vi "压力判定.vi"(7 "Result":refnum<vi>, 10 "判定参数":T2, 11 "XY曲线":cluster{"X":dbl[], "Y":dbl[]}[](array[cluster])) -> (2 "大小":i32, 3 "OK？":bool)   [LabVIEW 2020]
uses:
  Global_Variable/Global.vi
panel:
  in  "最大值判定":T1
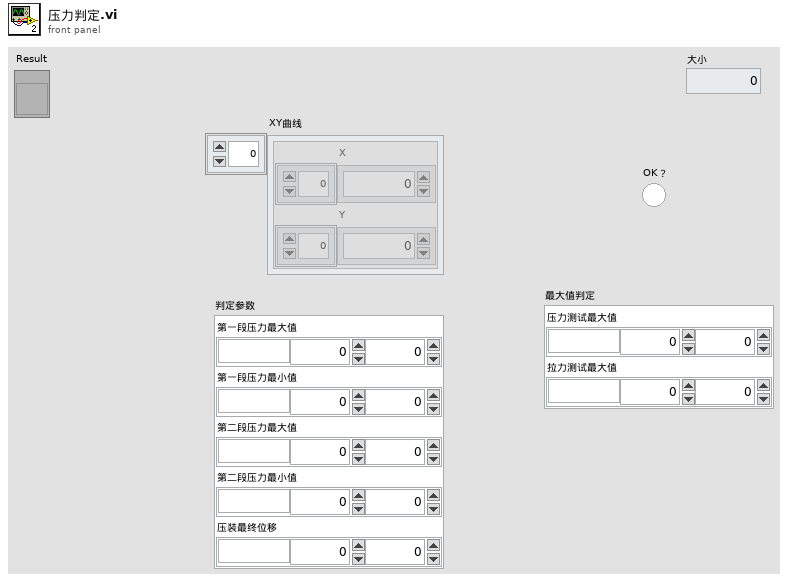
[diagram p1: front panel]
types:
  T1 = cluster{"压力测试最大值":cluster{"单位":string, "下限":dbl, "上限":dbl}, "拉力测试最大值":cluster{"单位":string, "下限":dbl, "上限":dbl}}
  T2 = cluster{"第一段压力最大值":cluster{"单位":string, "下限":dbl, "上限":dbl}, "第一段压力最小值":cluster{"单位":string, "下限":dbl, "上限":dbl}, "第二段压力最大值":cluster{"单位":string, "下限":dbl, "上限":dbl}, "第二段压力最小值":cluster{"单位":string, "下限":dbl, "上限":dbl}, "压装最终位移":cluster{"单位":string, "下限":dbl, "上限":dbl}}
  T3 = cluster{"第一段判定框位移":cluster{"单位":string, "下限":dbl, "上限":dbl}, "第一段判定框压力":cluster{"单位":string, "下限":dbl, "上限":dbl}, "低二段判定框位移":cluster{"单位":string, "下限":dbl, "上限":dbl}, "第二段判定框压力":cluster{"单位":string, "下限":dbl, "上限":dbl}}
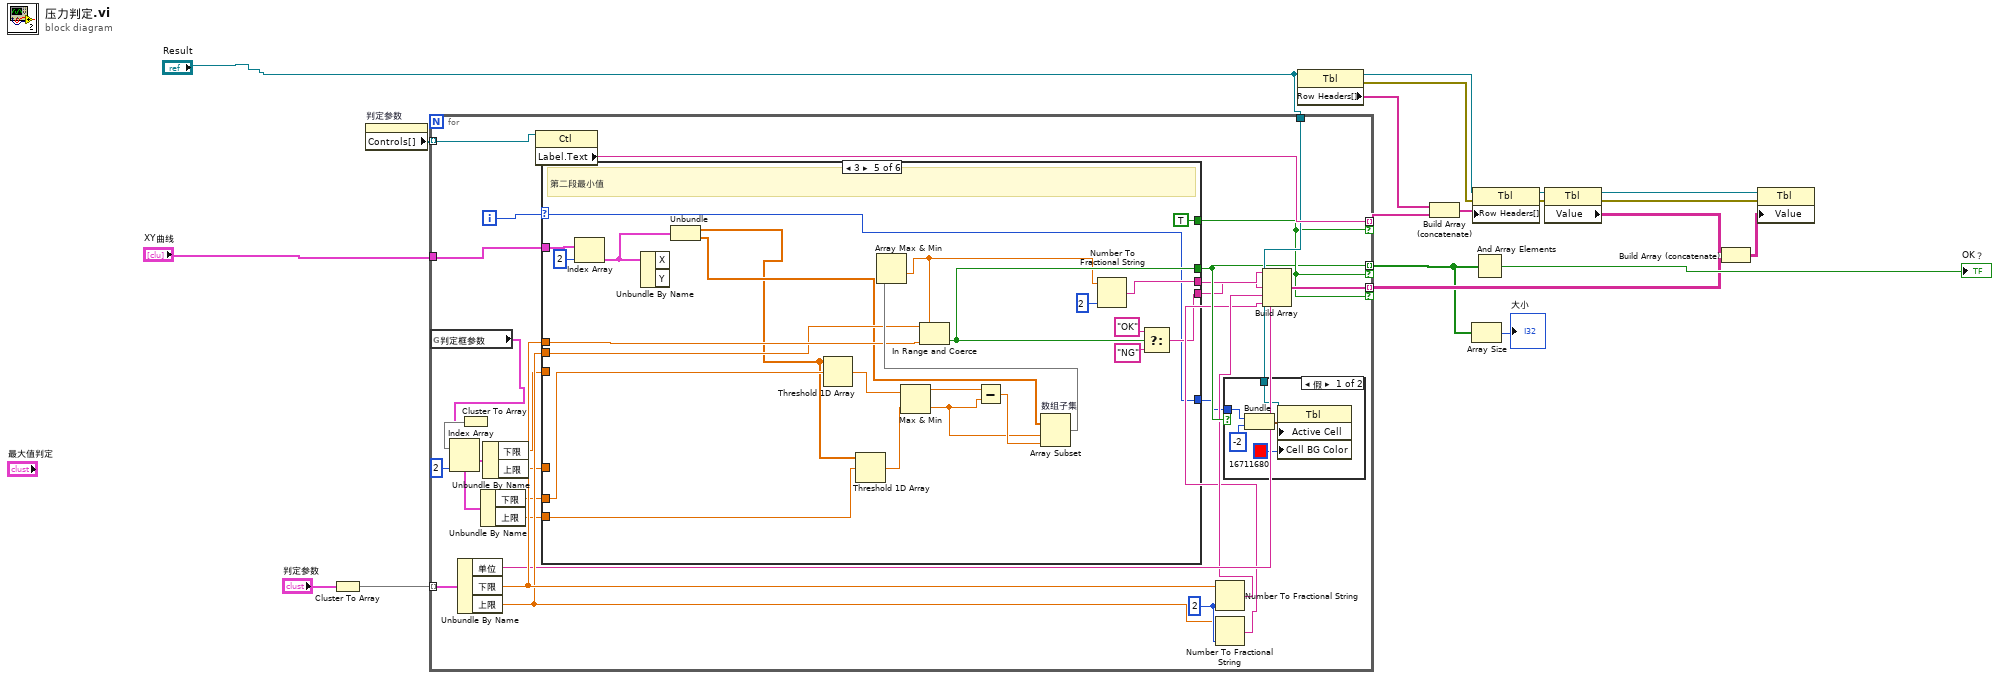
[diagram p0: block diagram]
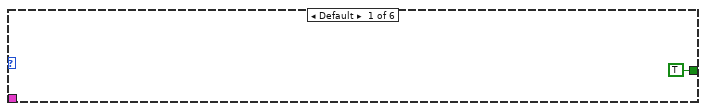
[diagram p3: hidden frame]
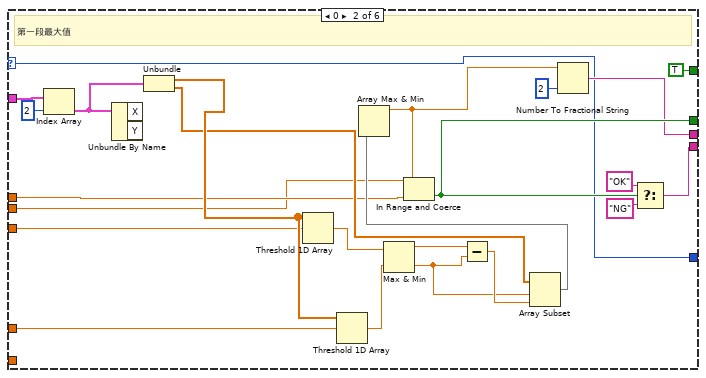
[diagram p4: hidden frame]
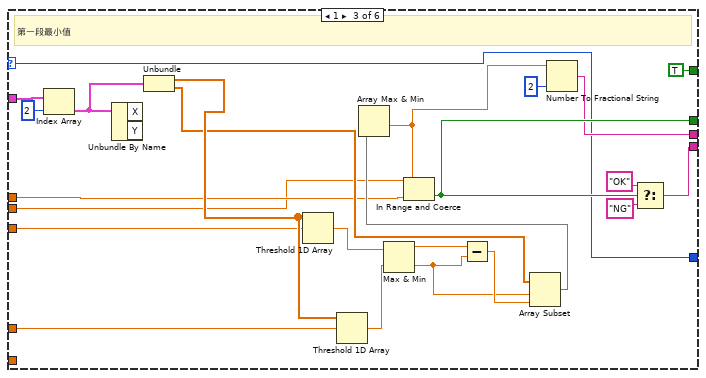
[diagram p5: hidden frame]
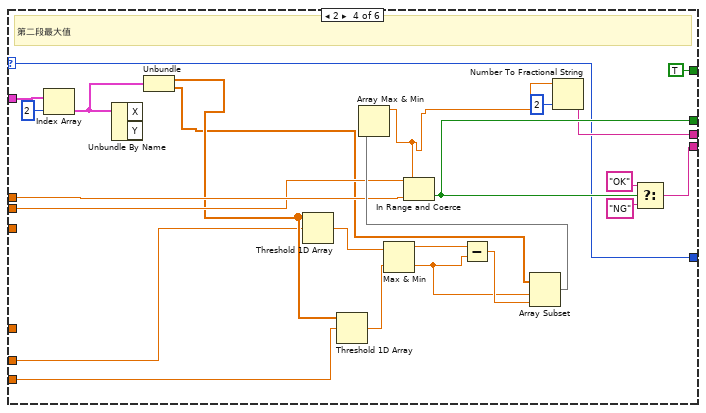
[diagram p6: hidden frame]
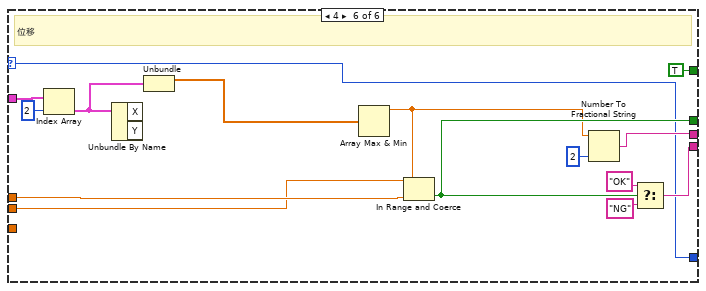
[diagram p7: hidden frame]
diagram:
  n1 = Cluster To Array(cluster="判定参数") -> (array=w20:cluster{"单位":string, "下限":dbl, "上限":dbl}[])
  n2 = property on="判定参数" class="Clust (严格)"() -> ("Controls[]"=w18:refnum<vi>[])  [unwired: 2 in, 2 out]
  n3 = for {
    tunnel: w20 -> [w47] mode=indexing
    tunnel: w18 -> [w45] mode=indexing
    tunnel: "XY曲线" -> [w44]
    tunnel: [w36] -> w2 mode=indexing if=w37
    tunnel: [w40] -> w4 mode=indexing if=w37
    tunnel: [w39] -> w6 mode=indexing if=w37
    tunnel: "Result" -> [w38]
    i -> [w46]
    w43 = i16 2 ("精度(6)")
    n4 = global read "Global.vi" "判定框参数"() -> (w26:T3)
    n5 = Unbundle By Name(w47) -> ("单位"=w34:string, "下限"=w42:dbl, "上限"=w41:dbl)
    n6 = Cluster To Array(cluster=w26) -> (array=w30:cluster{"单位":string, "下限":dbl, "上限":dbl}[])
    n7 = Index Array(array=w30, index #2=2 ("索引")) -> (element #1=w29:cluster{"单位":string, "下限":dbl, "上限":dbl}, element #2=w23:cluster{"单位":string, "下限":dbl, "上限":dbl})  [unwired: 1 in]
    n8 = Unbundle By Name(w23) -> ("下限"=w22:dbl, "上限"=w21:dbl)
    n9 = Unbundle By Name(w29) -> ("下限"=w28:dbl, "上限"=w27:dbl)
    n10 = property class="Ctl"(reference=w45) -> ("Label.Text"=w39:string)  [unwired: 1 in, 2 out]
    n11 = case shown="3" w46 {
      selector: w46 -> [_ w58 w82 w110 w134 w154]
      tunnel: w44 -> [_ w77 w101 w125 w149 w164]
      tunnel: [_ w74 w98 w122 w146 w161] -> w33
      tunnel: [_ w73 w97 w121 w145 w160] -> w36
      tunnel: w42 -> [_ w57 w81 w108 w132 w152]
      tunnel: w41 -> [_ w56 w80 w107 w131 w151]
      tunnel: [TRUE TRUE TRUE TRUE TRUE TRUE] -> w37
      tunnel: [_ w59 w83 w111 w135 w156] -> w35
      tunnel: [_ w58 w82 w110 w134 w154] -> w25
      tunnel: w28 -> [_ w55 w79 _ _ _]
      tunnel: w27 -> [_ w54 w78 _ _ _]
      tunnel: w22 -> [_ _ _ w103 w130 _]
      tunnel: w21 -> [_ _ _ w102 w129 _]
      frame Default {
      }
      frame 0 {
        # "第一段最大值"
        n12 = Index Array(array=w77, index=2 ("索引")) -> (element=w68:cluster{"X":dbl[], "Y":dbl[]})
        n13 = Unbundle By Name(w68) -> ()  [unwired: 2 out]
        n14 = Unbundle(w68) -> ("X"=w67:dbl[], "Y"=w64:dbl[])
        n15 = Threshold 1D Array(2:w55, 3:w67) -> (0:w71:dbl)  [unwired: 1 in]
        n16 = Threshold 1D Array(2:w54, 3:w67) -> (0:w70:dbl)  [unwired: 1 in]
        n17 = Max & Min(x=w71, y=w70) -> (max(x,y)=w69:dbl, min(x,y)=w65:dbl)
        n18 = Subtract(x=w69, y=w65) -> (x-y=w66:dbl)
        n19 = Array Subset(array=w64, index=w65, length=w66) -> (w63:dbl[])
        n20 = Array Max & Min(array=w63) -> (max value=w60:dbl)  [unwired: 3 out]
        n21 = In Range and Coerce(upper limit=w56, x=w60, lower limit=w57) -> (In Range?=w73:bool)  [unwired: 1 out]
        n22 = Number To Fractional String(number=w60, precision (6)=i16 2 ("精度(6)")) -> (F-format string=w59:string)  [unwired: 2 in]
        n23 = Select(t="OK", s=w73, f="NG") -> (s? t:f=w74:string)
      }
      frame 1 {
        # "第一段最小值"
        n24 = Index Array(array=w101, index=2 ("索引")) -> (element=w92:cluster{"X":dbl[], "Y":dbl[]})
        n25 = Unbundle By Name(w92) -> ()  [unwired: 2 out]
        n26 = Unbundle(w92) -> ("X"=w91:dbl[], "Y"=w88:dbl[])
        n27 = Threshold 1D Array(2:w79, 3:w91) -> (0:w95:dbl)  [unwired: 1 in]
        n28 = Threshold 1D Array(2:w78, 3:w91) -> (0:w94:dbl)  [unwired: 1 in]
        n29 = Max & Min(x=w95, y=w94) -> (max(x,y)=w93:dbl, min(x,y)=w89:dbl)
        n30 = Subtract(x=w93, y=w89) -> (x-y=w90:dbl)
        n31 = Array Subset(array=w88, index=w89, length=w90) -> (w87:dbl[])
        n32 = Array Max & Min(array=w87) -> (min value=w84:dbl)  [unwired: 3 out]
        n33 = In Range and Coerce(upper limit=w80, x=w84, lower limit=w81) -> (In Range?=w97:bool)  [unwired: 1 out]
        n34 = Number To Fractional String(number=w84, precision (6)=i16 2 ("精度(6)")) -> (F-format string=w83:string)  [unwired: 2 in]
        n35 = Select(t="OK", s=w97, f="NG") -> (s? t:f=w98:string)
      }
      frame 2 {
        # "第二段最大值"
        n36 = Index Array(array=w125, index=2 ("索引")) -> (element=w116:cluster{"X":dbl[], "Y":dbl[]})
        n37 = Unbundle By Name(w116) -> ()  [unwired: 2 out]
        n38 = Unbundle(w116) -> ("X"=w105:dbl[], "Y"=w104:dbl[])
        n39 = Threshold 1D Array(2:w103, 3:w105) -> (0:w119:dbl)  [unwired: 1 in]
        n40 = Threshold 1D Array(2:w102, 3:w105) -> (0:w118:dbl)  [unwired: 1 in]
        n41 = Max & Min(x=w119, y=w118) -> (max(x,y)=w117:dbl, min(x,y)=w114:dbl)
        n42 = Subtract(x=w117, y=w114) -> (x-y=w115:dbl)
        n43 = Array Subset(array=w104, index=w114, length=w115) -> (w113:dbl[])
        n44 = Array Max & Min(array=w113) -> (max value=w106:dbl)  [unwired: 3 out]
        n45 = In Range and Coerce(upper limit=w107, x=w106, lower limit=w108) -> (In Range?=w121:bool)  [unwired: 1 out]
        n46 = Number To Fractional String(number=w106, precision (6)=i16 2 ("精度(6)")) -> (F-format string=w111:string)  [unwired: 2 in]
        n47 = Select(t="OK", s=w121, f="NG") -> (s? t:f=w122:string)
      }
      frame 3 {
        # "第二段最小值"
        n48 = Index Array(array=w149, index=2 ("索引")) -> (element=w140:cluster{"X":dbl[], "Y":dbl[]})
        n49 = Unbundle By Name(w140) -> ()  [unwired: 2 out]
        n50 = Unbundle(w140) -> ("X"=w126:dbl[], "Y"=w127:dbl[])
        n51 = Threshold 1D Array(2:w130, 3:w126) -> (0:w143:dbl)  [unwired: 1 in]
        n52 = Threshold 1D Array(2:w129, 3:w126) -> (0:w142:dbl)  [unwired: 1 in]
        n53 = Max & Min(x=w143, y=w142) -> (max(x,y)=w141:dbl, min(x,y)=w138:dbl)
        n54 = Subtract(x=w141, y=w138) -> (x-y=w139:dbl)
        n55 = Array Subset "数组子集"(array=w127, index=w138, length=w139) -> (w137:dbl[])
        n56 = Array Max & Min(array=w137) -> (min value=w128:dbl)  [unwired: 3 out]
        n57 = In Range and Coerce(upper limit=w131, x=w128, lower limit=w132) -> (In Range?=w145:bool)  [unwired: 1 out]
        n58 = Number To Fractional String(number=w128, precision (6)=i16 2 ("精度(6)")) -> (F-format string=w135:string)  [unwired: 2 in]
        n59 = Select(t="OK", s=w145, f="NG") -> (s? t:f=w146:string)
      }
      frame 4 {
        # "位移"
        n60 = Index Array(array=w164, index=2 ("索引")) -> (element=w158:cluster{"X":dbl[], "Y":dbl[]})
        n61 = Unbundle By Name(w158) -> ()  [unwired: 2 out]
        n62 = Unbundle(w158) -> ("X"=w150:dbl[])  [unwired: 1 out]
        n63 = Array Max & Min(array=w150) -> (max value=w155:dbl)  [unwired: 3 out]
        n64 = In Range and Coerce(upper limit=w151, x=w155, lower limit=w152) -> (In Range?=w160:bool)  [unwired: 1 out]
        n65 = Number To Fractional String(number=w155, precision (6)=i16 2 ("精度(6)")) -> (F-format string=w156:string)  [unwired: 2 in]
        n66 = Select(t="OK", s=w160, f="NG") -> (s? t:f=w161:string)
      }
    }
    n67 = Number To Fractional String(number=w42, precision (6)=w43) -> (F-format string=w32:string)  [unwired: 2 in]
    n68 = Number To Fractional String(number=w41, precision (6)=w43) -> (F-format string=w31:string)  [unwired: 2 in]
    n69 = case shown="假" w36 {
      tunnel: w38 -> [w52 _]
      tunnel: w25 -> [w48 _]
      frame False {
        n70 = Bundle(w48, -2) -> (w50:cluster{i32, i32})  [unwired: 1 in]
        n71 = property class="Tbl"(reference=w52, "Active Cell"=w50, "Cell BG Color"=u32 16711680 ("活动单元格:单元格背景色")) -> ()  [unwired: 1 in, 2 out]
      }
      frame True {
      }
    }
    n72 = Build Array(w35, w34, w33, w32, w31) -> (w40:string[])
  }
  n73 = property class="Tbl"(reference="Result") -> (reference out=w8:refnum<vi>, error out=w13:errorcluster, "Row Headers[]"=w5:string[])  [unwired: 1 in]
  n74 = Build Array (concatenate)(w5, w6) -> (w7:string[])
  n75 = Array Size(array=w2) -> (size(s)=→"大小":i32)
  n76 = property class="Tbl"(reference=w8, error in=w13, "Row Headers[]"=w7) -> (reference out=w9:refnum<vi>, error out=w12:errorcluster)
  n77 = And Array Elements(Boolean array=w2) -> (logical AND=→"OK？":bool)
  n78 = property class="Tbl"(reference=w9, error in=w12) -> (reference out=w10:refnum<vi>, error out=w11:errorcluster, "Value"=w14:string[][])
  n79 = Build Array (concatenate)(w14, w4) -> (w15:string[][])
  n80 = property class="Tbl"(reference=w10, error in=w11, "Value"=w15) -> ()  [unwired: 2 out]
